vi "rel_humid_molar_fract_2024.vi"(2 "Pressure [Pa]":dbl=101325.0, 3 "enhancement factor":dbl=1.00357, 4 "saturated vapor pressure [Pa]":dbl=2339.25, 5 "rel. humidity":dbl=0.5 format="%_5g") -> (0 "Xw > 1 !":bool, 1 "xw water mole fraction":dbl=0.011584510843819394 format="%.6f")   [LabVIEW 2016]
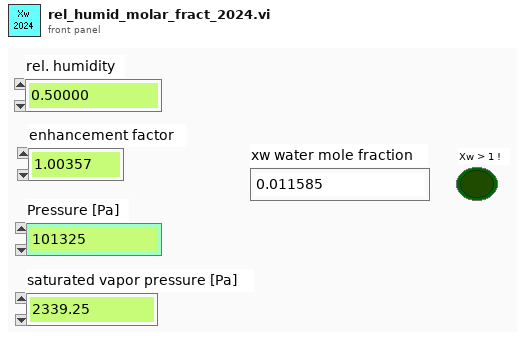
[diagram p1: front panel]
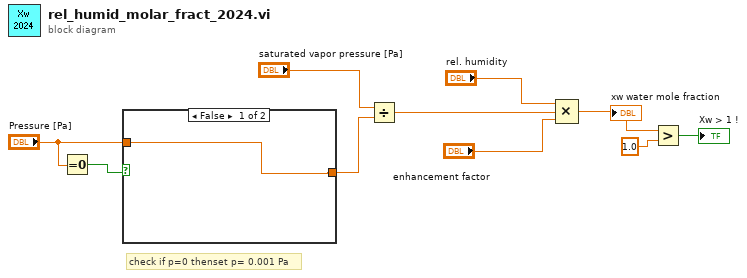
[diagram p0: block diagram]
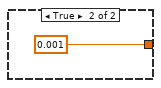
[diagram p2: hidden frame]
diagram:
  # "check if p=0 thenset p= 0.001 Pa"
  n1 = Equal To 0?(x="Pressure [Pa]") -> (x = 0?=w9:bool)
  n2 = case shown="False" w9 {
    tunnel: [w11 0.001] -> w8
    tunnel: "Pressure [Pa]" -> [w11 _]
    frame False {
    }
    frame True {
    }
  }
  n3 = Divide(x="saturated vapor pressure [Pa]", y=w8) -> (x/y=w6:dbl)
  n4 = Compound Arithmetic op=MULTIPLY("rel. humidity", w6, "enhancement factor") -> (w4:dbl)
  "xw water mole fraction" <- w4
  n5 = Greater?(x=w4, y=1.0) -> (0:→"Xw > 1 !":bool)
